vi "make_controls_available.vi"(0 "input cluster":T1, 1 "Make Available":bool) -> ()   [LabVIEW 2010]
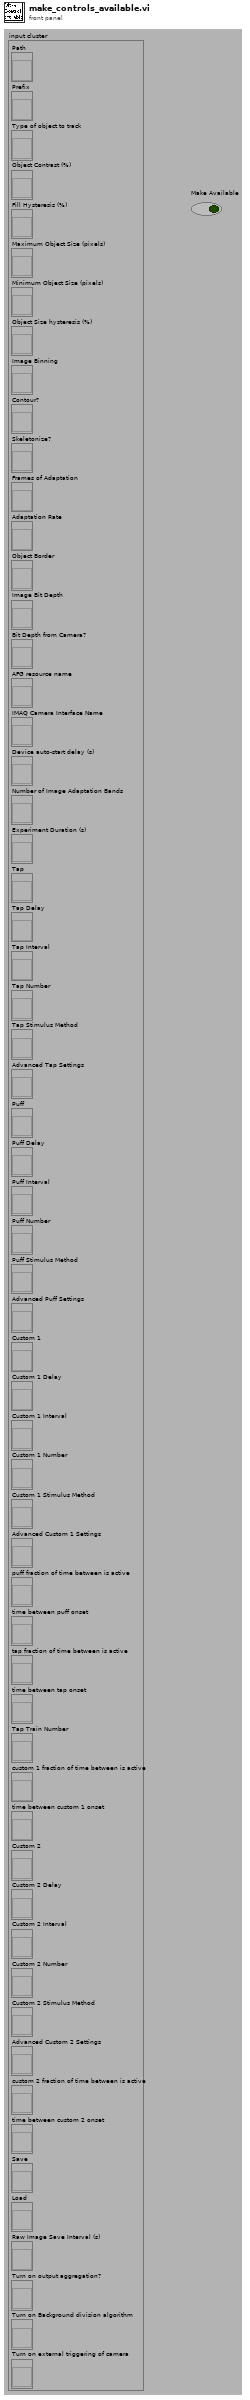
[diagram p1: front panel]
types:
  T1 = cluster{"Path":refnum<vi>, "Prefix":refnum<vi>, "Type of object to track":refnum<vi>, "Object Contrast (%)":refnum<vi>, "Fill Hysteresis (%)":refnum<vi>, "Maximum Object Size (pixels)":refnum<vi>, "Minimum Object Size (pixels)":refnum<vi>, "Object Size hysteresis (%)":refnum<vi>, "Image Binning":refnum<vi>, "Contour?":refnum<vi>, "Skeletonize?":refnum<vi>, "Frames of Adaptation":refnum<vi>, "Adaptation Rate":refnum<vi>, "Object Border":refnum<vi>, "Image Bit Depth":refnum<vi>, "Bit Depth from Camera?":refnum<vi>, "AFG resource name":refnum<vi>, "IMAQ Camera Interface Name":refnum<vi>, "Device auto-start delay (s)":refnum<vi>, "Number of Image Adaptation Bands":refnum<vi>, "Experiment Duration (s)":refnum<vi>, "Tap":refnum<vi>, "Tap Delay":refnum<vi>, "Tap Interval":refnum<vi>, "Tap Number":refnum<vi>, "Tap Stimulus Method":refnum<vi>, "Advanced Tap Settings":refnum<vi>, "Puff":refnum<vi>, "Puff Delay":refnum<vi>, "Puff Interval":refnum<vi>, "Puff Number":refnum<vi>, "Puff Stimulus Method":refnum<vi>, "Advanced Puff Settings":refnum<vi>, "Custom 1":refnum<vi>, "Custom 1 Delay":refnum<vi>, "Custom 1 Interval":refnum<vi>, "Custom 1 Number":refnum<vi>, "Custom 1 Stimulus Method":refnum<vi>, "Advanced Custom 1 Settings":refnum<vi>, "puff fraction of time between is active":refnum<vi>, "time between puff onset":refnum<vi>, "tap fraction of time between is active":refnum<vi>, "time between tap onset":refnum<vi>, "Tap Train Number":refnum<vi>, "custom 1 fraction of time between is active":refnum<vi>, "time between custom 1 onset":refnum<vi>, "Custom 2":refnum<vi>, "Custom 2 Delay":refnum<vi>, "Custom 2 Interval":refnum<vi>, "Custom 2 Number":refnum<vi>, "Custom 2 Stimulus Method":refnum<vi>, "Advanced Custom 2 Settings":refnum<vi>, "custom 2 fraction of time between is active":refnum<vi>, "time between custom 2 onset":refnum<vi>, "Save":refnum<vi>, "Load":refnum<vi>, "Raw Image Save Interval (s)":refnum<vi>, "Turn on output aggregation?":refnum<vi>, "Turn on Background division algorithm":refnum<vi>, "Turn on external triggering of camera":refnum<vi>}
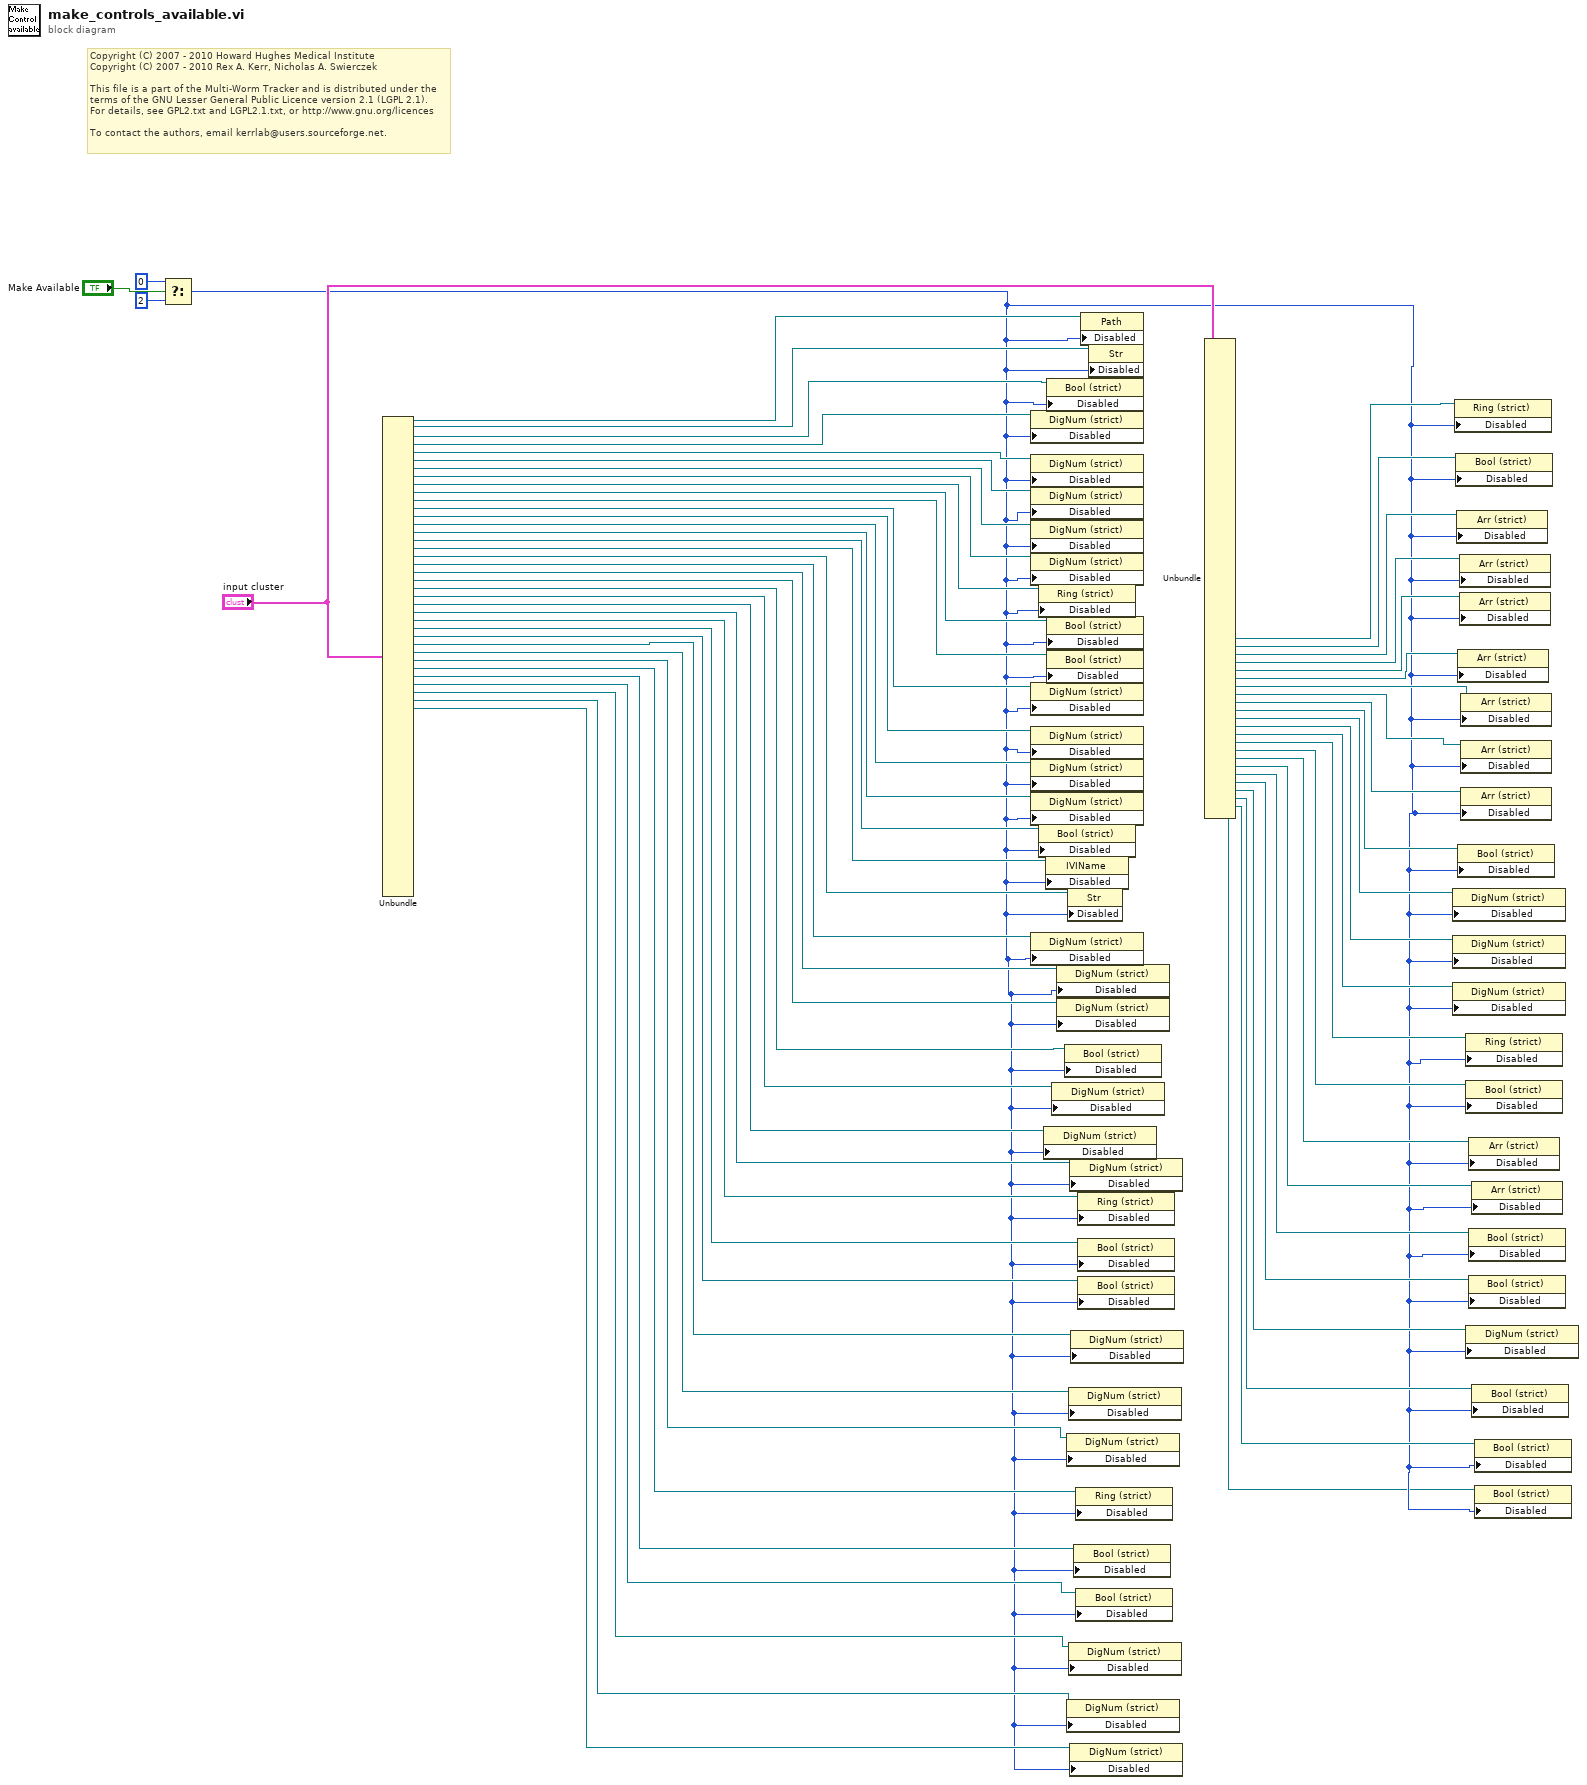
[diagram p0: block diagram]
diagram:
  # "Copyright (C) 2007 - 2010 Howard Hughes Medical Institute\nCopyright (C) 2007 - 2010 Rex A. Kerr, Nicholas A. Swierczek\n \nThis file is a part of the Multi-Worm Tracker and is distributed under the\nterms of the GNU Lesser General Public Licence version 2.1 (LGPL 2.1).\nFor details, see GPL2.txt and LGPL2.1.txt, or http://www.gnu.org/licences\n \nTo contact the authors, email kerrlab@users.sourceforge.net."
  n1 = Select(t=0, s="Make Available", f=2) -> (s? t:f=w2:i32)
  n2 = Unbundle("input cluster") -> ("Path"=w65:refnum<vi>, "Prefix"=w64:refnum<vi>, "Type of object to track"=w63:refnum<vi>, "Object Contrast (%)"=w62:refnum<vi>, "Fill Hysteresis (%)"=w61:refnum<vi>, "Maximum Object Size (pixels)"=w60:refnum<vi>, "Minimum Object Size (pixels)"=w59:refnum<vi>, "Object Size hysteresis (%)"=w58:refnum<vi>, "Image Binning"=w57:refnum<vi>, "Contour?"=w56:refnum<vi>, "Skeletonize?"=w55:refnum<vi>, "Frames of Adaptation"=w54:refnum<vi>, "Adaptation Rate"=w53:refnum<vi>, "Object Border"=w52:refnum<vi>, "Image Bit Depth"=w51:refnum<vi>, "Bit Depth from Camera?"=w50:refnum<vi>, "AFG resource name"=w49:refnum<vi>, "IMAQ Camera Interface Name"=w48:refnum<vi>, "Device auto-start delay (s)"=w47:refnum<vi>, "Number of Image Adaptation Bands"=w46:refnum<vi>, "Experiment Duration (s)"=w45:refnum<vi>, "Tap"=w44:refnum<vi>, "Tap Delay"=w43:refnum<vi>, "Tap Interval"=w42:refnum<vi>, "Tap Number"=w41:refnum<vi>, "Tap Stimulus Method"=w40:refnum<vi>, "Advanced Tap Settings"=w39:refnum<vi>, "Puff"=w38:refnum<vi>, "Puff Delay"=w37:refnum<vi>, "Puff Interval"=w36:refnum<vi>, "Puff Number"=w35:refnum<vi>, "Puff Stimulus Method"=w34:refnum<vi>, "Advanced Puff Settings"=w33:refnum<vi>, "Custom 1"=w32:refnum<vi>, "Custom 1 Delay"=w31:refnum<vi>, "Custom 1 Interval"=w30:refnum<vi>, "Custom 1 Number"=w29:refnum<vi>)  [unwired: 23 out]
  n3 = property class="DigNum (strict)"(reference=w62, "Disabled"=w2) -> ()  [unwired: 1 in, 2 out]
  n4 = property class="DigNum (strict)"(reference=w61, "Disabled"=w2) -> ()  [unwired: 1 in, 2 out]
  n5 = property class="DigNum (strict)"(reference=w60, "Disabled"=w2) -> ()  [unwired: 1 in, 2 out]
  n6 = property class="DigNum (strict)"(reference=w59, "Disabled"=w2) -> ()  [unwired: 1 in, 2 out]
  n7 = property class="DigNum (strict)"(reference=w58, "Disabled"=w2) -> ()  [unwired: 1 in, 2 out]
  n8 = property class="DigNum (strict)"(reference=w54, "Disabled"=w2) -> ()  [unwired: 1 in, 2 out]
  n9 = property class="DigNum (strict)"(reference=w53, "Disabled"=w2) -> ()  [unwired: 1 in, 2 out]
  n10 = property class="DigNum (strict)"(reference=w52, "Disabled"=w2) -> ()  [unwired: 1 in, 2 out]
  n11 = property class="DigNum (strict)"(reference=w51, "Disabled"=w2) -> ()  [unwired: 1 in, 2 out]
  n12 = property class="DigNum (strict)"(reference=w47, "Disabled"=w2) -> ()  [unwired: 1 in, 2 out]
  n13 = property class="Ring (strict)"(reference=w57, "Disabled"=w2) -> ()  [unwired: 1 in, 2 out]
  n14 = property class="Bool (strict)"(reference=w50, "Disabled"=w2) -> ()  [unwired: 1 in, 2 out]
  n15 = property class="DigNum (strict)"(reference=w42, "Disabled"=w2) -> ()  [unwired: 1 in, 2 out]
  n16 = property class="IVIName"(reference=w49, "Disabled"=w2) -> ()  [unwired: 1 in, 2 out]
  n17 = property class="Bool (strict)"(reference=w63, "Disabled"=w2) -> ()  [unwired: 1 in, 2 out]
  n18 = property class="Bool (strict)"(reference=w56, "Disabled"=w2) -> ()  [unwired: 1 in, 2 out]
  n19 = property class="Bool (strict)"(reference=w55, "Disabled"=w2) -> ()  [unwired: 1 in, 2 out]
  n20 = property class="DigNum (strict)"(reference=w43, "Disabled"=w2) -> ()  [unwired: 1 in, 2 out]
  n21 = property class="DigNum (strict)"(reference=w46, "Disabled"=w2) -> ()  [unwired: 1 in, 2 out]
  n22 = property class="DigNum (strict)"(reference=w45, "Disabled"=w2) -> ()  [unwired: 1 in, 2 out]
  n23 = property class="Bool (strict)"(reference=w44, "Disabled"=w2) -> ()  [unwired: 1 in, 2 out]
  n24 = property class="DigNum (strict)"(reference=w35, "Disabled"=w2) -> ()  [unwired: 1 in, 2 out]
  n25 = property class="DigNum (strict)"(reference=w30, "Disabled"=w2) -> ()  [unwired: 1 in, 2 out]
  n26 = property class="Str"(reference=w48, "Disabled"=w2) -> ()  [unwired: 1 in, 2 out]
  n27 = property class="DigNum (strict)"(reference=w36, "Disabled"=w2) -> ()  [unwired: 1 in, 2 out]
  n28 = property class="DigNum (strict)"(reference=w31, "Disabled"=w2) -> ()  [unwired: 1 in, 2 out]
  n29 = property class="DigNum (strict)"(reference=w41, "Disabled"=w2) -> ()  [unwired: 1 in, 2 out]
  n30 = property class="DigNum (strict)"(reference=w29, "Disabled"=w2) -> ()  [unwired: 1 in, 2 out]
  n31 = property class="DigNum (strict)"(reference=w37, "Disabled"=w2) -> ()  [unwired: 1 in, 2 out]
  n32 = property class="Bool (strict)"(reference=w33, "Disabled"=w2) -> ()  [unwired: 1 in, 2 out]
  n33 = property class="Ring (strict)"(reference=w34, "Disabled"=w2) -> ()  [unwired: 1 in, 2 out]
  n34 = property class="Bool (strict)"(reference=w32, "Disabled"=w2) -> ()  [unwired: 1 in, 2 out]
  n35 = property class="Ring (strict)"(reference=w40, "Disabled"=w2) -> ()  [unwired: 1 in, 2 out]
  n36 = property class="Bool (strict)"(reference=w39, "Disabled"=w2) -> ()  [unwired: 1 in, 2 out]
  n37 = property class="Bool (strict)"(reference=w38, "Disabled"=w2) -> ()  [unwired: 1 in, 2 out]
  n38 = property class="Path"(reference=w65, "Disabled"=w2) -> ()  [unwired: 1 in, 2 out]
  n39 = property class="Str"(reference=w64, "Disabled"=w2) -> ()  [unwired: 1 in, 2 out]
  n40 = Unbundle("input cluster") -> ("Custom 1 Stimulus Method"=w28:refnum<vi>, "Advanced Custom 1 Settings"=w27:refnum<vi>, "puff fraction of time between is active"=w26:refnum<vi>, "time between puff onset"=w25:refnum<vi>, "tap fraction of time between is active"=w24:refnum<vi>, "time between tap onset"=w23:refnum<vi>, "Tap Train Number"=w22:refnum<vi>, "custom 1 fraction of time between is active"=w21:refnum<vi>, "time between custom 1 onset"=w20:refnum<vi>, "Custom 2"=w16:refnum<vi>, "Custom 2 Delay"=w15:refnum<vi>, "Custom 2 Interval"=w14:refnum<vi>, "Custom 2 Number"=w13:refnum<vi>, "Custom 2 Stimulus Method"=w12:refnum<vi>, "Advanced Custom 2 Settings"=w11:refnum<vi>, "custom 2 fraction of time between is active"=w10:refnum<vi>, "time between custom 2 onset"=w9:refnum<vi>, "Save"=w8:refnum<vi>, "Load"=w7:refnum<vi>, "Raw Image Save Interval (s)"=w6:refnum<vi>, "Turn on output aggregation?"=w5:refnum<vi>, "Turn on Background division algorithm"=w4:refnum<vi>, "Turn on external triggering of camera"=w1:refnum<vi>)  [unwired: 37 out]
  n41 = property class="DigNum (strict)"(reference=w15, "Disabled"=w2) -> ()  [unwired: 1 in, 2 out]
  n42 = property class="DigNum (strict)"(reference=w14, "Disabled"=w2) -> ()  [unwired: 1 in, 2 out]
  n43 = property class="DigNum (strict)"(reference=w13, "Disabled"=w2) -> ()  [unwired: 1 in, 2 out]
  n44 = property class="Ring (strict)"(reference=w28, "Disabled"=w2) -> ()  [unwired: 1 in, 2 out]
  n45 = property class="Bool (strict)"(reference=w27, "Disabled"=w2) -> ()  [unwired: 1 in, 2 out]
  n46 = property class="Arr (strict)"(reference=w26, "Disabled"=w2) -> ()  [unwired: 1 in, 2 out]
  n47 = property class="Arr (strict)"(reference=w23, "Disabled"=w2) -> ()  [unwired: 1 in, 2 out]
  n48 = property class="Bool (strict)"(reference=w16, "Disabled"=w2) -> ()  [unwired: 1 in, 2 out]
  n49 = property class="Arr (strict)"(reference=w25, "Disabled"=w2) -> ()  [unwired: 1 in, 2 out]
  n50 = property class="Arr (strict)"(reference=w24, "Disabled"=w2) -> ()  [unwired: 1 in, 2 out]
  n51 = property class="Arr (strict)"(reference=w22, "Disabled"=w2) -> ()  [unwired: 1 in, 2 out]
  n52 = property class="Arr (strict)"(reference=w21, "Disabled"=w2) -> ()  [unwired: 1 in, 2 out]
  n53 = property class="Arr (strict)"(reference=w20, "Disabled"=w2) -> ()  [unwired: 1 in, 2 out]
  n54 = property class="Ring (strict)"(reference=w12, "Disabled"=w2) -> ()  [unwired: 1 in, 2 out]
  n55 = property class="Bool (strict)"(reference=w11, "Disabled"=w2) -> ()  [unwired: 1 in, 2 out]
  n56 = property class="DigNum (strict)"(reference=w6, "Disabled"=w2) -> ()  [unwired: 1 in, 2 out]
  n57 = property class="Arr (strict)"(reference=w10, "Disabled"=w2) -> ()  [unwired: 1 in, 2 out]
  n58 = property class="Bool (strict)"(reference=w8, "Disabled"=w2) -> ()  [unwired: 1 in, 2 out]
  n59 = property class="Bool (strict)"(reference=w7, "Disabled"=w2) -> ()  [unwired: 1 in, 2 out]
  n60 = property class="Arr (strict)"(reference=w9, "Disabled"=w2) -> ()  [unwired: 1 in, 2 out]
  n61 = property class="Bool (strict)"(reference=w5, "Disabled"=w2) -> ()  [unwired: 1 in, 2 out]
  n62 = property class="Bool (strict)"(reference=w4, "Disabled"=w2) -> ()  [unwired: 1 in, 2 out]
  n63 = property class="Bool (strict)"(reference=w1, "Disabled"=w2) -> ()  [unwired: 1 in, 2 out]
